vi "Auto_Drive (2).vi"(10 "Target":dbl format="%#_13g", 11 "Drive Effort":dbl=0.3) -> ()   [LabVIEW 2016]
uses:
  <vilib>/Rock Robotics/WPI/SafetyOutput/WPI_SafetyOutputConfigMenu.ctl
  Global 2.vi
panel:
  in  "kP":dbl=1.0 format="%#_13g"
  in  "kD":dbl format="%#_13g"
  in  "Scaling Factor":dbl=16.0 format="%#_13g"
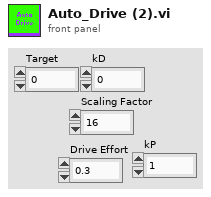
[diagram p1: front panel]
types:
  T1 = typedef "WPI_SafetyOutputConfigMenu.ctl" = enum16{"Enable", "Disable"}
  T2 = typedef "WPI_MotorControlDeviceRef.ctl" = cluster{"DeviceStatus":errorcluster, "Type":T3, "PWM":cluster{"PWM Channel":T4, "DeadBand":T5}, "CAN":cluster{"Device Number":u8, "SetOutput VI Ref":variant, "GetOutput VI Ref":variant, "Enable VI Ref":variant, "Disable VI Ref":variant, "Data":variant}, "Invert":bool}
  T3 = typedef "WPI_MotorControlType.ctl" = enum16{"PWM", "CAN"}
  T4 = typedef "FPGA_DIOPWMChannel.ctl" = enum8{"PWM 0", "PWM 1", "PWM 2", "PWM 3", "PWM 4", "PWM 5", "PWM 6", "PWM 7", "PWM 8", "PWM 9", "PWM MXP 0", "PWM MXP 1", "PWM MXP 2", "PWM MXP 3", "PWM MXP 4", "PWM MXP 5", "PWM MXP 6", "PWM MXP 7", "PWM MXP 8", "PWM MXP 9", "Invalid"}
  T5 = typedef "WPI_PWMDeadband.ctl" = cluster{"Name":string, "maxPositivePwm":i32, "minPositivePwm":i32, "centerPwm":i32, "maxNegativePwm":i32, "minNegativePwm":i32, "angularRange":u16}
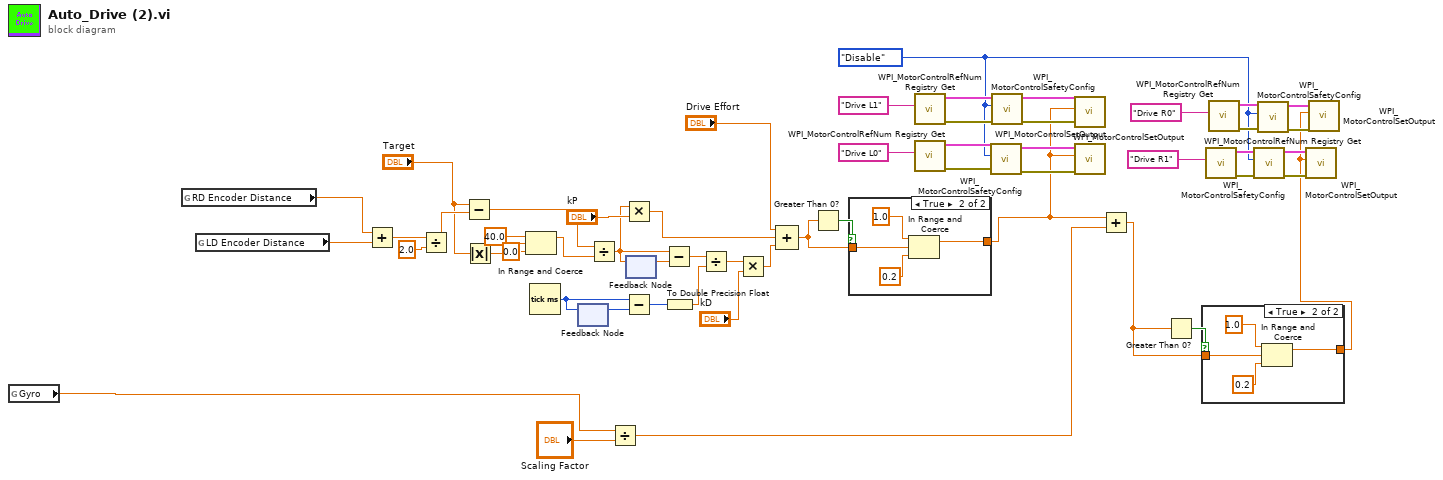
[diagram p0: block diagram]
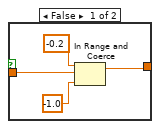
[diagram p2: hidden frame]
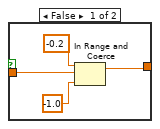
[diagram p3: hidden frame]
diagram:
  w34 = WPI_SafetyOutputConfigMenu."Disable" ("mode")
  n1 = global read "Global 2.vi" "Gyro"() -> (w31:dbl)
  n2 = global read "Global 2.vi" "RD Encoder Distance"() -> (w8:dbl)
  n3 = global read "Global 2.vi" "LD Encoder Distance"() -> (w9:dbl)
  n4 = Add(x=w8, y=w9) -> (x+y=w29:dbl)
  n5 = Divide(x=w29, y=2.0) -> (x/y=w27:dbl)
  n6 = Subtract(x="Target", y=w27) -> (x-y=w15:dbl)
  n7 = Absolute Value(x="Target") -> (abs(x)=w6:dbl)
  n8 = In Range and Coerce(upper limit=40.0, x=w6, lower limit=0.0) -> (coerced(x)=w4:dbl)  [unwired: 1 out]
  n9 = Tick Count (ms)() -> (millisecond timer value=w23:u32)
  n10 = feedback #1() -> (w24:u32)  [unwired: 1 in]
  n11 = feedback-in #1(w23) -> ()
  n12 = Divide(x=w15, y=w4) -> (x/y=w14:dbl)
  n13 = Divide(x=w31, y="Scaling Factor") -> (x/y=w32:dbl)
  n14 = Multiply(x=w14, y="kP") -> (x*y=w17:dbl)
  n15 = Subtract(x=w23, y=w24) -> (x-y=w21:u32)
  n16 = feedback #2() -> (w25:dbl)  [unwired: 1 in]
  n17 = feedback-in #2(w14) -> ()
  n18 = Subtract(x=w14, y=w25) -> (x-y=w22:dbl)
  n19 = To Double Precision Float(number=w21) -> (double precision float=w20:dbl)
  n20 = Divide(x=w22, y=w20) -> (x/y=w19:dbl)
  n21 = Multiply(x=w19, y="kD") -> (x*y=w16:dbl)
  n22 = Compound Arithmetic op=ADD("Drive Effort", w17, w16) -> (w12:dbl)
  n23 = Greater Than 0?(x=w12) -> (x > 0?=w13:bool)
  n24 = case shown="True" w13 {
    tunnel: [w55 w60] -> w11
    tunnel: w12 -> [w56 w59]
    frame False {
      n25 = In Range and Coerce(upper limit=-0.2, x=w56, lower limit=-1.0) -> (coerced(x)=w55:dbl)  [unwired: 1 out]
    }
    frame True {
      n26 = In Range and Coerce(upper limit=1.0, x=w59, lower limit=0.2) -> (coerced(x)=w60:dbl)  [unwired: 1 out]
    }
  }
  n27 = call <vilib>:"WPI_MotorControlRefNum Registry Get.vi"("refnum name"="Drive L1") -> ("error out"=w49:errorcluster, "MotorControlDevRef"=w50:T2)  [unwired: 9 in]
  n28 = call <vilib>:"WPI_MotorControlRefNum Registry Get.vi"("refnum name"="Drive L0") -> ("error out"=w45:errorcluster, "MotorControlDevRef"=w46:T2)  [unwired: 9 in]
  n29 = call <vilib>:"WPI_MotorControlSafetyConfig.vi"("error in (no error)"=w45, "mode"=w34, "MotorControlDevRef"=w46) -> ("error out"=w43:errorcluster, "MotorControlDevRef"=w44:T2)  [unwired: 7 in]
  n30 = call <vilib>:"WPI_MotorControlSafetyConfig.vi"("error in (no error)"=w49, "mode"=w34, "MotorControlDevRef"=w50) -> ("error out"=w47:errorcluster, "MotorControlDevRef"=w48:T2)  [unwired: 7 in]
  n31 = call <vilib>:"WPI_MotorControlSetOutput.vi"("error in (no error)"=w47, "Output"=w11, "MotorControlDevRef"=w48) -> ()  [unwired: 6 in, 3 out]
  n32 = call <vilib>:"WPI_MotorControlSetOutput.vi"("error in (no error)"=w43, "Output"=w11, "MotorControlDevRef"=w44) -> ()  [unwired: 6 in, 3 out]
  n33 = Add(x=w11, y=w32) -> (x+y=w1:dbl)
  n34 = Greater Than 0?(x=w1) -> (x > 0?=w3:bool)
  n35 = case shown="True" w3 {
    tunnel: [w63 w68] -> w2
    tunnel: w1 -> [w64 w67]
    frame False {
      n36 = In Range and Coerce(upper limit=-0.2, x=w64, lower limit=-1.0) -> (coerced(x)=w63:dbl)  [unwired: 1 out]
    }
    frame True {
      n37 = In Range and Coerce(upper limit=1.0, x=w67, lower limit=0.2) -> (coerced(x)=w68:dbl)  [unwired: 1 out]
    }
  }
  n38 = call <vilib>:"WPI_MotorControlRefNum Registry Get.vi"("refnum name"="Drive R1") -> ("error out"=w37:errorcluster, "MotorControlDevRef"=w38:T2)  [unwired: 9 in]
  n39 = call <vilib>:"WPI_MotorControlRefNum Registry Get.vi"("refnum name"="Drive R0") -> ("error out"=w41:errorcluster, "MotorControlDevRef"=w42:T2)  [unwired: 9 in]
  n40 = call <vilib>:"WPI_MotorControlSafetyConfig.vi"("error in (no error)"=w37, "mode"=w34, "MotorControlDevRef"=w38) -> ("error out"=w36:errorcluster, "MotorControlDevRef"=w35:T2)  [unwired: 7 in]
  n41 = call <vilib>:"WPI_MotorControlSafetyConfig.vi"("error in (no error)"=w41, "mode"=w34, "MotorControlDevRef"=w42) -> ("error out"=w40:errorcluster, "MotorControlDevRef"=w39:T2)  [unwired: 7 in]
  n42 = call <vilib>:"WPI_MotorControlSetOutput.vi"("error in (no error)"=w36, "Output"=w2, "MotorControlDevRef"=w35) -> ()  [unwired: 6 in, 3 out]
  n43 = call <vilib>:"WPI_MotorControlSetOutput.vi"("error in (no error)"=w40, "Output"=w2, "MotorControlDevRef"=w39) -> ()  [unwired: 6 in, 3 out]
